vi "Réponse Opérateur.vi"(8 "errin":errorcluster, 11 "expression régulière":string) -> (0 "errout":errorcluster, 1 "toute l'expression":string, 3 "ArrsurErr":bool)   [LabVIEW 2020]
doc: "Vérifie le retour d'une saisie en fonction d'une expression régulière"
uses:
  <vilib>/regexp/Match Regular Expression.xnode
panel:
  out "out":string
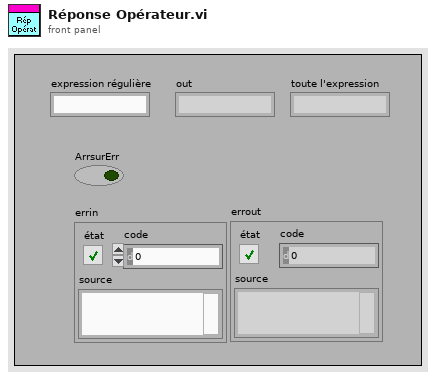
[diagram p1: front panel]
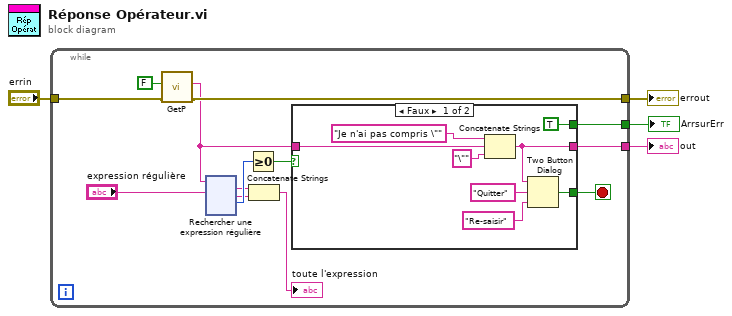
[diagram p0: block diagram]
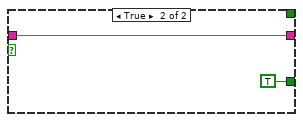
[diagram p2: hidden frame]
diagram:
  n1 = while {
    tunnel: "errin" -> [w8]
    tunnel: [w17] -> w4
    tunnel: [w7] -> w2
    tunnel: [w15] -> w1
    stop <- w16 stop-if-true
    n2 = call "GetP.vi"("errin"=w8, "Pédale ON?"=FALSE) -> ("errout"=w7:errorcluster, "Data out"=w6:string)  [unwired: 8 in]
    n3 = xnode "Rechercher une expression régulière"("chaîne en entrée"=w6, "expression régulière"="expression régulière") -> ("toute l'expression"=w11:string, "après la correspondance"=w10:string, "offset après correspondance"=w12:i32)  [unwired: 4 in, 2 out]
    n4 = Greater Or Equal To 0?(x=w12) -> (x >= 0?=w14:bool)
    n5 = Concatenate Strings(w11, w10) -> (→"toute l'expression":string)
    n6 = case shown="Faux" w14 {
      tunnel: [TRUE _] -> w17
      tunnel: [w137 TRUE ("T button?")] -> w16
      tunnel: w6 -> [w133 w140]
      tunnel: [w132 w140] -> w15
      frame False {
        n7 = Concatenate Strings("Je n'ai pas compris \"" ("message"), w133, "\"" ("chaîne")) -> (w132:string)
        n8 = Two Button Dialog(message=w132, 1:"Re-saisir" ("Nom du bouton V (\"OK\")"), 2:"Quitter" ("Nom du bouton F (\"Annuler\")")) -> (T button?=w137:bool)
      }
      frame True {
      }
    }
  }
  "ArrsurErr" <- w4
  "errout" <- w2
  "out" <- w1
